vi "final Vi_2.vi"() -> ()   [LabVIEW 2018]
uses:
  <vilib>/Utility/file.llb/Read Delimited Spreadsheet (string).vi
  <vilib>/Utility/file.llb/Read Delimited Spreadsheet (DBL).vi
  <vilib>/Analysis/3filter.llb/Equi-Ripple BandPass (DBL).vi
  <vilib>/Analysis/NI_AALBase.lvlib
  <vilib>/Analysis/NI_AAL_SigProc.lvlib
panel:
  out "Array 2":dbl[](array[numeric])
  out "我們計算的RR":cluster{i32[], dbl[]}(graph)
  out "Array":dbl[](array[numeric])
  in  "threshold":dbl=10000.0 format="%0.2f"
  out "Locations":dbl[](array[numeric])
  in  "filter higher  stop freq":dbl(slide)=0.4094594594594595 scale=0.4..0.5
  out "平均心跳/分鐘":dbl
  out "?":bool
  out "RMSSD(ms)":dbl
  out "HR":cluster{i32[], dbl[]}[](graph)
  out "Mean R-R interval":dbl
  out "RR":cluster{dbl[], dbl[]}(graph)
  in  "filter lower stop freq":dbl(slide)=0.032972972972972976 scale=0.0..0.1
  out "Band filter":cluster{dbl[], "Filtered X":dbl[]}[](graph)
  out "Origin ECG":cluster{dbl[], i32[]}(graph)
  # "RMSSD越大，\n表示副交感神經作用越強"
  # "一般正常心跳約為50~100下/分鐘"
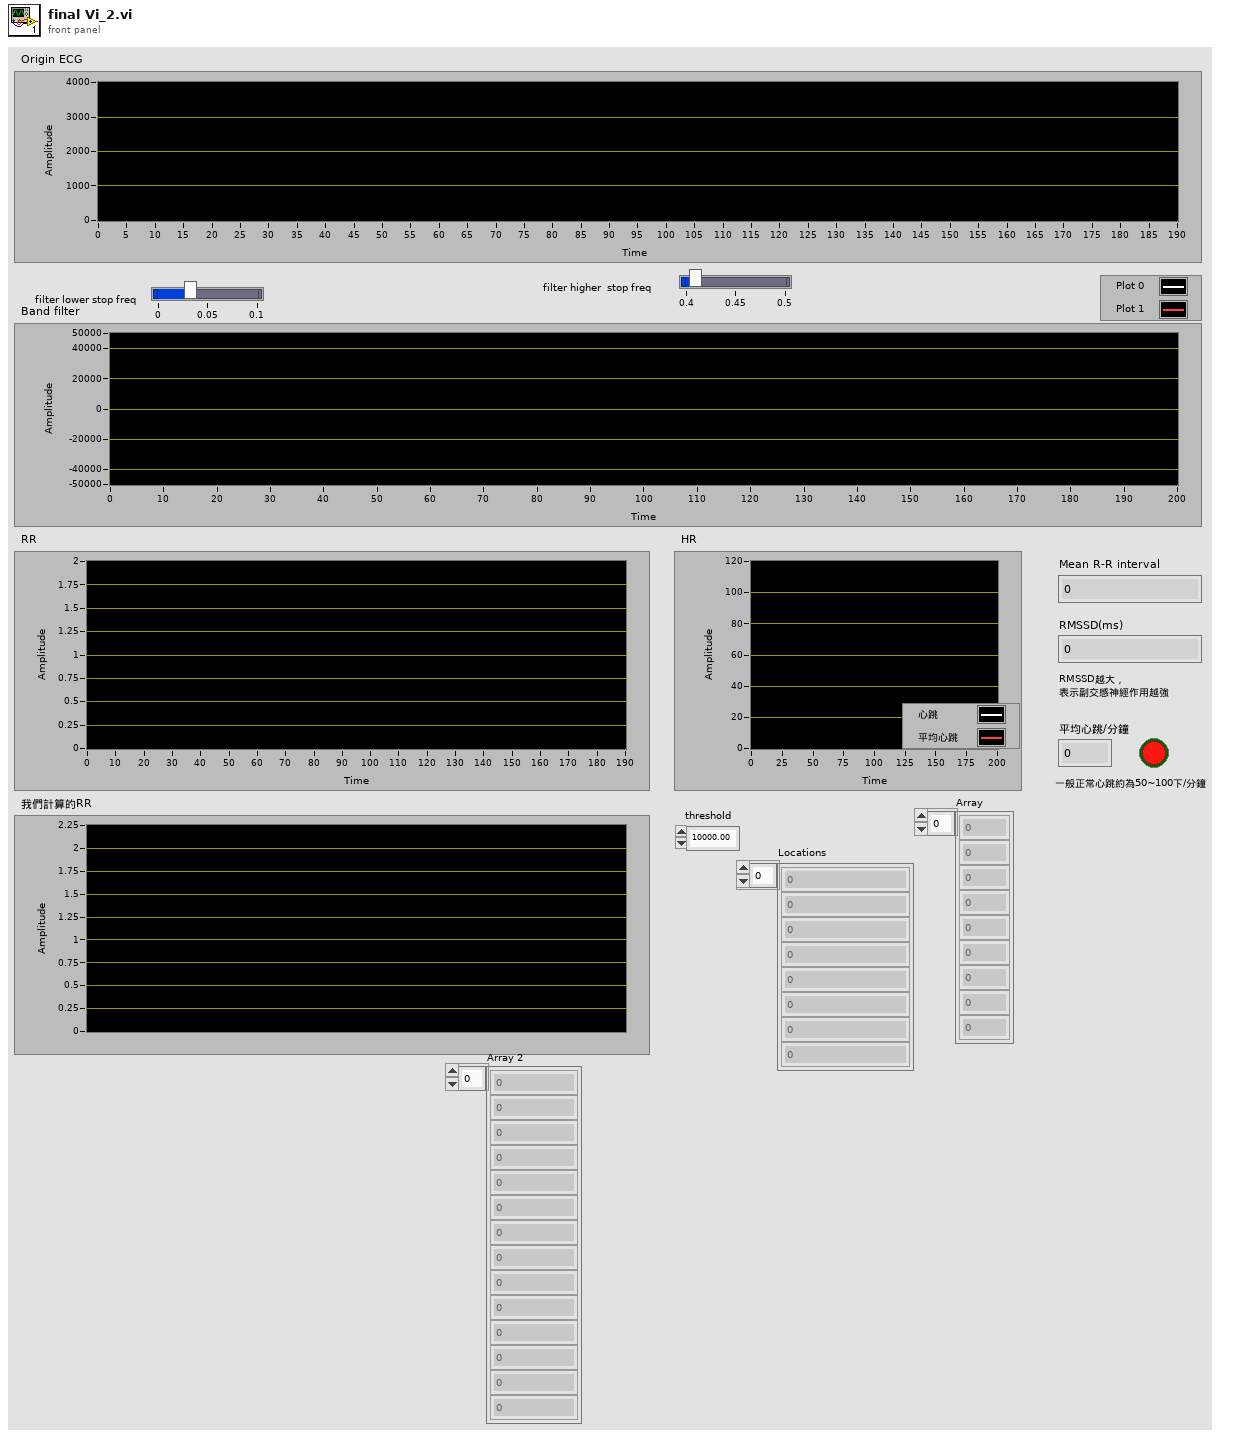
[diagram p1: front panel]
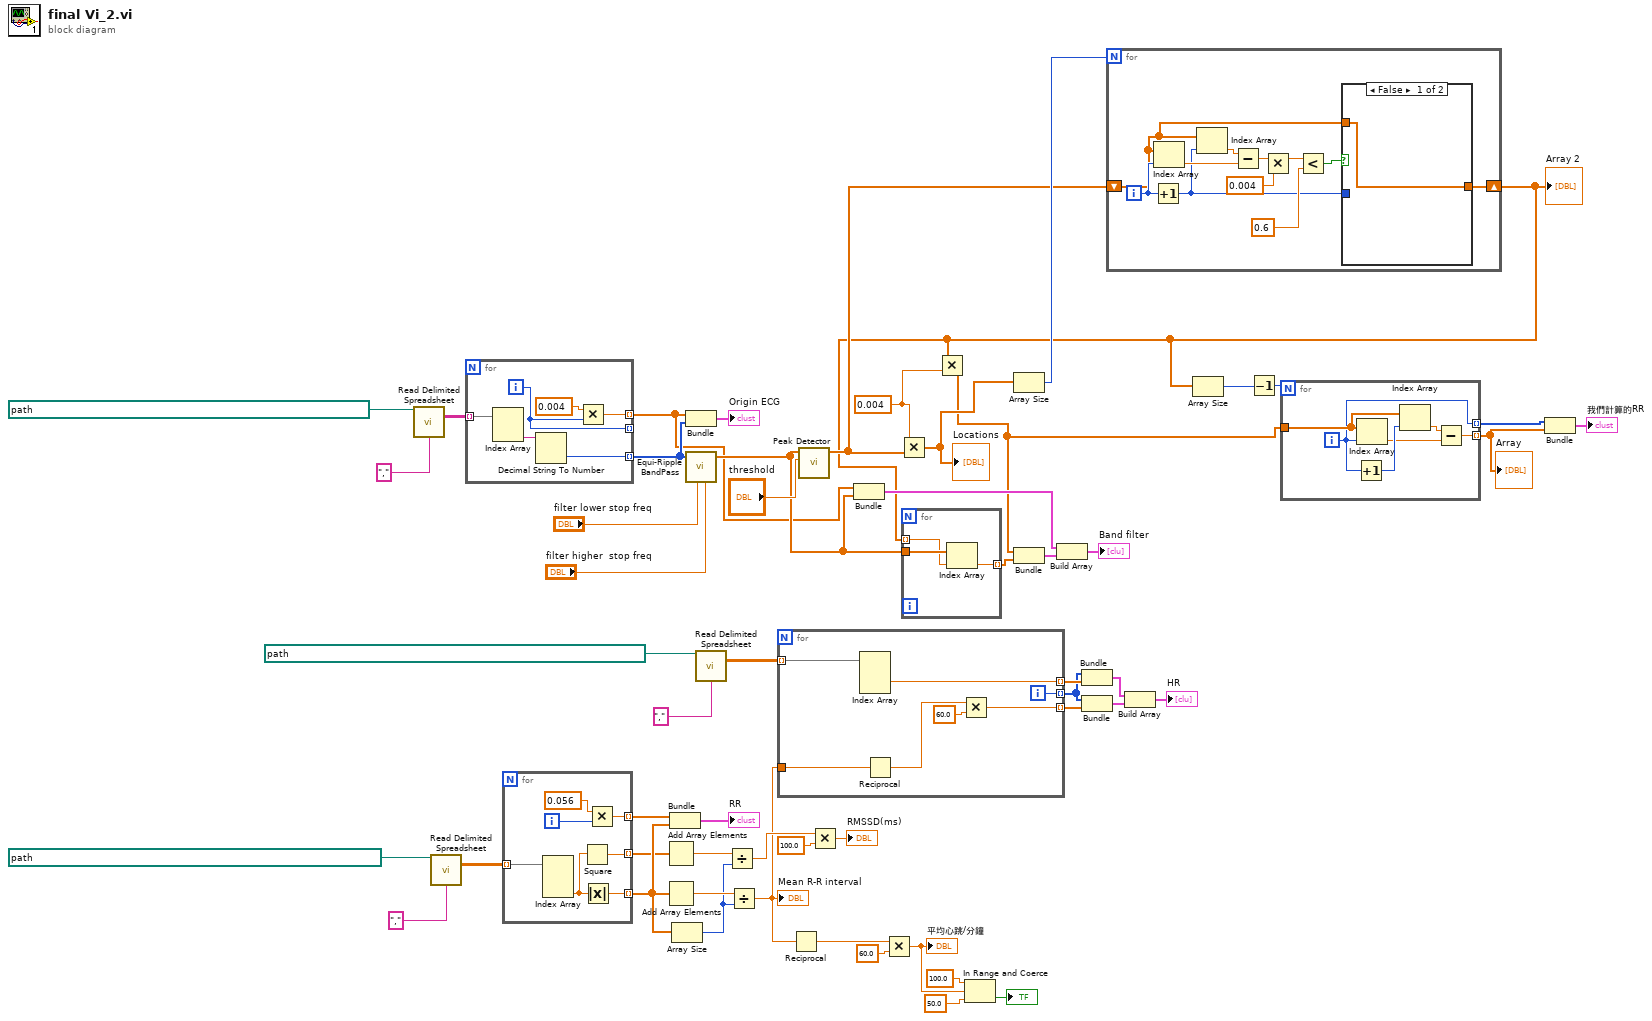
[diagram p0: block diagram]
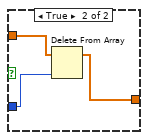
[diagram p2: hidden frame]
diagram:
  w5 = 0.004 ("y")
  n1 = call-poly <vilib>:"Read Delimited Spreadsheet.vi"("file path (dialog if empty)"=path "D:/Documents/生醫儀表/data/2019_05_25__16_08_04_ECG.csv", "delimiter (\\t)"="," ("delimiter (\\t)")) -> ("all rows"=w53:string[][])  [unwired: 8 in, 5 out]
  n2 = call-poly <vilib>:"Read Delimited Spreadsheet.vi"("file path (dialog if empty)"=path "D:/Documents/生醫儀表/data/2019_05_25__16_08_04_BR_RR.csv", "delimiter (\\t)"="," ("delimiter (\\t)")) -> ("all rows"=w50:dbl[][])  [unwired: 8 in, 5 out]
  n3 = for {
    tunnel: w53 -> [w60] mode=indexing
    tunnel: [w59] -> w17 mode=indexing
    tunnel: [w57] -> w10 mode=indexing
    tunnel: [w55] -> _ mode=indexing
    i -> [w55]
    n4 = Index Array(array=w60) -> (element #2=w56:string)  [unwired: 2 in, 1 out]
    n5 = Decimal String To Number(string=w56) -> (number=w59:i32)  [unwired: 2 in, 1 out]
    n6 = Multiply(x=0.004 ("y"), y=w55) -> (x*y=w57:dbl)
  }
  n7 = for {
    tunnel: w50 -> [w67] mode=indexing
    tunnel: [w64] -> w48 mode=indexing
    tunnel: [w63] -> w44 mode=indexing
    tunnel: [w61] -> w34 mode=indexing
    i -> [w66]
    n8 = Index Array(array=w67) -> (element #3=w62:dbl)  [unwired: 3 in, 2 out]
    n9 = Square(x=w62) -> (x^2=w61:dbl)
    n10 = Absolute Value(x=w62) -> (abs(x)=w63:dbl)
    n11 = Multiply(x=0.056 ("y"), y=w66) -> (x*y=w64:dbl)
  }
  n12 = Add Array Elements(numeric array=w34) -> (sum=w33:dbl)
  n13 = Add Array Elements(numeric array=w44) -> (sum=w45:dbl)
  n14 = Bundle(w48, w44) -> (→"RR":cluster{dbl[], dbl[]})  [unwired: 1 in]
  n15 = Array Size(array=w44) -> (size(s)=w32:i32)
  n16 = Bundle(w10, w17) -> (→"Origin ECG":cluster{dbl[], i32[]})  [unwired: 1 in]
  n17 = call-poly <vilib>:"Equi-Ripple BandPass.vi"("X"=w17, "lower stop freq"="filter lower stop freq", "higher stop freq"="filter higher  stop freq") -> ("Filtered X"=w11:dbl[])  [unwired: 5 in, 1 out]
  n18 = call-poly <vilib>:"Read Delimited Spreadsheet.vi"("file path (dialog if empty)"=path "D:/Documents/生醫儀表/data/2019_05_25__16_08_04_General.csv", "delimiter (\\t)"="," ("delimiter (\\t)")) -> ("all rows"=w41:dbl[][])  [unwired: 8 in, 5 out]
  n19 = Divide(x=w33, y=w32) -> (x/y=w31:dbl)
  n20 = Divide(x=w45, y=w32) -> (x/y=w26:dbl)
  "Mean R-R interval" <- w26
  n21 = for {
    tunnel: w41 -> [w74] mode=indexing
    tunnel: [w73] -> w40 mode=indexing
    tunnel: [w72] -> w39 mode=indexing
    tunnel: w26 -> [w71]
    tunnel: [w68] -> w35 mode=indexing
    i -> [w72]
    n22 = Index Array(array=w74) -> (element #2=w73:dbl)  [unwired: 3 in, 2 out]
    n23 = Reciprocal(x=w71) -> (1/x=w70:dbl)
    n24 = Multiply(x=w70, y=60.0) -> (x*y=w68:dbl)
  }
  n25 = Reciprocal(x=w26) -> (1/x=w28:dbl)
  n26 = call <vilib>:"Peak Detector.vi"("threshold"="threshold", "X"=w11) -> ("Locations"=w6:dbl[])  [unwired: 5 in, 4 out]
  n27 = Multiply(x=w31, y=100.0) -> (x*y=→"RMSSD(ms)":dbl)
  n28 = Bundle(w10, "Filtered X"=w11) -> (w15:cluster{dbl[], "Filtered X":dbl[]})  [unwired: 1 in]
  n29 = Multiply(x=w28, y=60.0) -> (x*y=w25:dbl)
  "平均心跳/分鐘" <- w25
  n30 = Multiply(x=w5, y=w6) -> (x*y=w7:dbl[])
  "Locations" <- w7
  n31 = In Range and Coerce(upper limit=100.0, x=w25, lower limit=50.0) -> (In Range?=→"?":bool)  [unwired: 1 out]
  n32 = Array Size(array=w7) -> (size(s)=w8:i32)
  n33 = Bundle(w39, w40) -> (w38:cluster{i32[], dbl[]})  [unwired: 1 in]
  n34 = Bundle(w39, w35) -> (w36:cluster{i32[], dbl[]})  [unwired: 1 in]
  n35 = for {
    N: w8 -> [_]
    shift-right: [w77] -> w1
    shift-left: w6 -> [w79]
    i -> [w85]
    n36 = Increment(x=w85) -> (x+1=w78:i32)
    n37 = Index Array(array=w79, index=w85) -> (element=w83:dbl)
    n38 = Index Array(array=w79, index=w78) -> (element=w84:dbl)
    n39 = Subtract(x=w84, y=w83) -> (x-y=w82:dbl)
    n40 = Multiply(x=w82, y=0.004) -> (x*y=w76:dbl)
    n41 = Less?(x=w76, y=0.6) -> (x < y?=w80:bool)
    n42 = case shown="False" w80 {
      tunnel: w79 -> [w86 w89]
      tunnel: w78 -> [_ w88]
      tunnel: [w86 w87] -> w77
      frame False {
      }
      frame True {
        n43 = Delete From Array(array=w89, index=w88) -> (array with subset deleted=w87:dbl[])  [unwired: 1 in, 1 out]
      }
    }
  }
  "Array 2" <- w1
  n44 = for {
    tunnel: w1 -> [w91] mode=indexing
    tunnel: w11 -> [w92]
    tunnel: [w90] -> w13 mode=indexing
    n45 = Index Array(array=w92, index=w91) -> (element=w90:dbl)
  }
  n46 = Multiply(x=w1, y=w5) -> (x*y=w4:dbl[])
  n47 = Bundle(w4, w13) -> (w12:cluster{dbl[], dbl[]})  [unwired: 1 in]
  n48 = Build Array(w15, w12) -> (→"Band filter":cluster{dbl[], "Filtered X":dbl[]}[])
  n49 = Build Array(w38, w36) -> (→"HR":cluster{i32[], dbl[]}[])
  n50 = Array Size(array=w1) -> (size(s)=w3:i32)
  n51 = Decrement(x=w3) -> (x-1=w2:i32)
  n52 = for {
    N: w2 -> [_]
    tunnel: w4 -> [w98]
    tunnel: [w94] -> w9 mode=indexing
    tunnel: [w93] -> w18 mode=indexing
    i -> [w93]
    n53 = Increment(x=w93) -> (x+1=w97:i32)
    n54 = Index Array(array=w98, index=w93) -> (element=w95:dbl)
    n55 = Index Array(array=w98, index=w97) -> (element=w96:dbl)
    n56 = Subtract(x=w96, y=w95) -> (x-y=w94:dbl)
  }
  "Array" <- w9
  n57 = Bundle(w18, w9) -> (→"我們計算的RR":cluster{i32[], dbl[]})  [unwired: 1 in]
